vi "Byte Buffer.Write.Typed Double Array.vi"(0 "Byte Buffer in":refnum<class "Byte Buffer.lvclass">, 1 "data type":T1, 5 "buffer in":dbl[](array[numeric]), 7 "count":i64, 9 "buffer offset":u64, 11 "error in (no error)":errorcluster) -> (4 "Byte Buffer out":refnum<class "Byte Buffer.lvclass">, 6 "buffer out":dbl[](array[numeric]), 10 "new buffer offset":u64, 15 "error out":errorcluster)   [LabVIEW 2016, in "VeriStand Data.lvlib" / "Byte Buffer.lvclass"]
doc: "Reads <B>count</B> number of elements from the provided double float <B>buffer</B> and writes them to the <B>Byte Buffer</B> at the specified <B>buffer offset</B> and converted to the specified <B>data type</B>."
uses:
  Byte Buffer.lvclass
  Typedefs/Typedefs.Data Types.ctl
  Byte Buffer.lvclass/Byte Buffer.ctl
  Byte Buffer.Write (1D Boolean).vi
  Type Conversion/Type Conversion.From Double.Subset (1D Boolean).vi
  Byte Buffer.Write (1D SGL).vi
  Type Conversion/Type Conversion.From Double.Subset (1D SGL).vi
  Byte Buffer.Write (1D DBL).vi
  Byte Buffer.Write (1D I8).vi
  Type Conversion/Type Conversion.From Double.Subset (1D I8).vi
  Byte Buffer.Write (1D I16).vi
  Type Conversion/Type Conversion.From Double.Subset (1D I16).vi
  Byte Buffer.Write (1D I32).vi
  Type Conversion/Type Conversion.From Double.Subset (1D I32).vi
  Byte Buffer.Write (1D I64).vi
  Type Conversion/Type Conversion.From Double.Subset (1D I64).vi
  Byte Buffer.Write (1D U8).vi
  Type Conversion/Type Conversion.From Double.Subset (1D U8).vi
  Byte Buffer.Write (1D U16).vi
  Type Conversion/Type Conversion.From Double.Subset (1D U16).vi
  Byte Buffer.Write (1D U32).vi
  Type Conversion/Type Conversion.From Double.Subset (1D U32).vi
  Byte Buffer.Write (1D U64).vi
  Type Conversion/Type Conversion.From Double.Subset (1D U64).vi
  Byte Buffer.Write (String).vi
  Type Conversion/Type Conversion.From Double.vi
  Type Conversion/Type Conversion.From Double (1D Boolean).vi
  Type Conversion/Type Conversion.From Double (1D SGL).vi
  Type Conversion/Type Conversion.From Double (1D I8).vi
  Type Conversion/Type Conversion.From Double (1D I16).vi
  Type Conversion/Type Conversion.From Double (1D I32).vi
  Type Conversion/Type Conversion.From Double (1D I64).vi
  Type Conversion/Type Conversion.From Double (1D U8).vi
  Type Conversion/Type Conversion.From Double (1D U16).vi
  Type Conversion/Type Conversion.From Double (1D U32).vi
  Type Conversion/Type Conversion.From Double (1D U64).vi
  Byte Buffer.Subset.Set.vi
  Byte Buffer.Get Buffer Pointer.vi
  Byte Buffer.Get Buffer Size.vi
  Memory Management/Memory Management.MoveByteBlock.Read (String).vi
  Memory Management/Memory Management.Handle Return.vi
  Byte Buffer.Get Byte Order.vi
  VeriStand Data.lvlib
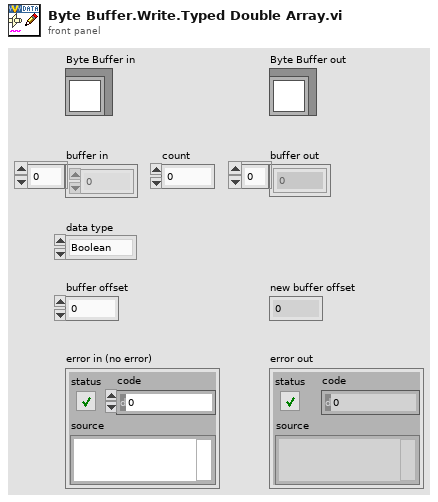
[diagram p1: front panel]
types:
  T1 = typedef "VeriStand Data.lvlib/Typedefs.Data Types.ctl" = enum16{"Boolean", "Single", "Double", "I8", "I16", "I32", "I64", "U8", "U16", "U32", "U64"}
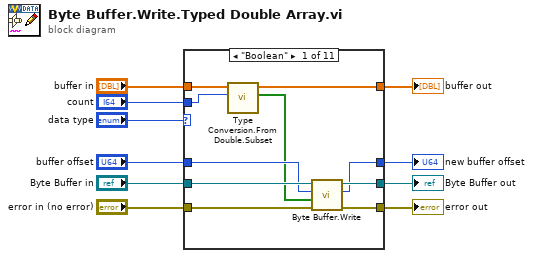
[diagram p0: block diagram]
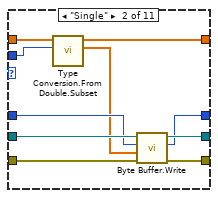
[diagram p2: hidden frame]
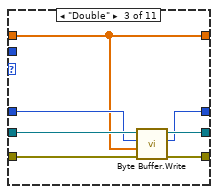
[diagram p3: hidden frame]
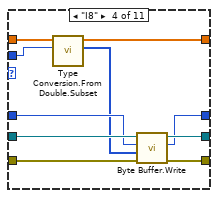
[diagram p4: hidden frame]
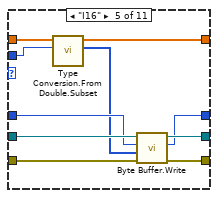
[diagram p5: hidden frame]
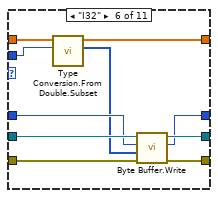
[diagram p6: hidden frame]
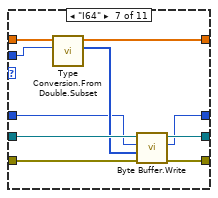
[diagram p7: hidden frame]
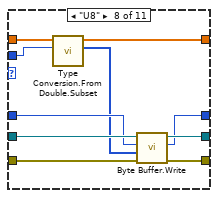
[diagram p8: hidden frame]
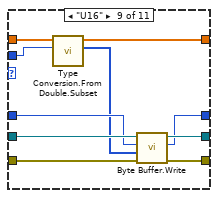
[diagram p9: hidden frame]
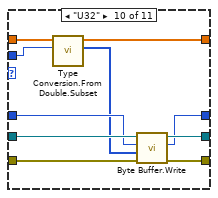
[diagram p10: hidden frame]
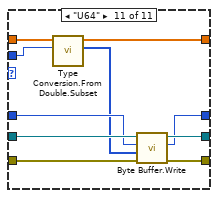
[diagram p11: hidden frame]
diagram:
  n1 = case shown="\"Boolean\"" "data type" {
    tunnel: "buffer in" -> [w20 w30 w32 w47 w57 w67 w77 w87 w97 w107 w117]
    tunnel: "buffer offset" -> [w17 w27 w35 w44 w54 w64 w69 w84 w94 w104 w114]
    tunnel: "Byte Buffer in" -> [w19 w29 w37 w46 w56 w66 w76 w86 w96 w106 w116]
    tunnel: [w18 w28 w36 w45 w55 w65 w75 w85 w95 w105 w115] -> w10
    tunnel: "error in (no error)" -> [w16 w26 w34 w43 w53 w63 w74 w83 w93 w103 w113]
    tunnel: [w15 w25 w33 w42 w52 w62 w73 w82 w92 w102 w112] -> w8
    tunnel: [w14 w24 w32 w41 w51 w61 w72 w81 w91 w101 w111] -> w6
    tunnel: "count" -> [w13 w23 _ w40 w50 w60 w71 w80 w90 w100 w110]
    tunnel: [w11 w21 w31 w38 w48 w58 w68 w78 w88 w98 w108] -> w2
    frame "Boolean" {
      n2 = call-poly "Type Conversion.From Double.Subset.vi"("count"=w13, "values in"=w20) -> ("converted values out"=w12:bool[], "values out"=w14:dbl[])  [unwired: 8 in]
      n3 = call-poly "Byte Buffer.Write.vi"("error in (no error)"=w16, "values"=w12, "buffer offset"=w17, "Byte Buffer in"=w19) -> ("error out"=w15:errorcluster, "new buffer offset"=w11:u64, "Byte Buffer out"=w18:refnum<class "Byte Buffer.lvclass">)  [unwired: 5 in]
    }
    frame "Single" {
      n4 = call-poly "Type Conversion.From Double.Subset.vi"("count"=w23, "values in"=w30) -> ("converted values out"=w22:sgl[], "values out"=w24:dbl[])  [unwired: 8 in]
      n5 = call-poly "Byte Buffer.Write.vi"("error in (no error)"=w26, "values"=w22, "buffer offset"=w27, "Byte Buffer in"=w29) -> ("error out"=w25:errorcluster, "new buffer offset"=w21:u64, "Byte Buffer out"=w28:refnum<class "Byte Buffer.lvclass">)  [unwired: 5 in]
    }
    frame "Double" {
      n6 = call-poly "Byte Buffer.Write.vi"("error in (no error)"=w34, "values"=w32, "buffer offset"=w35, "Byte Buffer in"=w37) -> ("error out"=w33:errorcluster, "new buffer offset"=w31:u64, "Byte Buffer out"=w36:refnum<class "Byte Buffer.lvclass">)  [unwired: 5 in]
    }
    frame "I8" {
      n7 = call-poly "Type Conversion.From Double.Subset.vi"("count"=w40, "values in"=w47) -> ("converted values out"=w39:i8[], "values out"=w41:dbl[])  [unwired: 8 in]
      n8 = call-poly "Byte Buffer.Write.vi"("error in (no error)"=w43, "values"=w39, "buffer offset"=w44, "Byte Buffer in"=w46) -> ("error out"=w42:errorcluster, "new buffer offset"=w38:u64, "Byte Buffer out"=w45:refnum<class "Byte Buffer.lvclass">)  [unwired: 5 in]
    }
    frame "I16" {
      n9 = call-poly "Type Conversion.From Double.Subset.vi"("count"=w50, "values in"=w57) -> ("converted values out"=w49:i16[], "values out"=w51:dbl[])  [unwired: 8 in]
      n10 = call-poly "Byte Buffer.Write.vi"("error in (no error)"=w53, "values"=w49, "buffer offset"=w54, "Byte Buffer in"=w56) -> ("error out"=w52:errorcluster, "new buffer offset"=w48:u64, "Byte Buffer out"=w55:refnum<class "Byte Buffer.lvclass">)  [unwired: 5 in]
    }
    frame "I32" {
      n11 = call-poly "Type Conversion.From Double.Subset.vi"("count"=w60, "values in"=w67) -> ("converted values out"=w59:i32[], "values out"=w61:dbl[])  [unwired: 8 in]
      n12 = call-poly "Byte Buffer.Write.vi"("error in (no error)"=w63, "values"=w59, "buffer offset"=w64, "Byte Buffer in"=w66) -> ("error out"=w62:errorcluster, "new buffer offset"=w58:u64, "Byte Buffer out"=w65:refnum<class "Byte Buffer.lvclass">)  [unwired: 5 in]
    }
    frame "I64" {
      n13 = call-poly "Type Conversion.From Double.Subset.vi"("count"=w71, "values in"=w77) -> ("converted values out"=w70:i64[], "values out"=w72:dbl[])  [unwired: 8 in]
      n14 = call-poly "Byte Buffer.Write.vi"("error in (no error)"=w74, "values"=w70, "buffer offset"=w69, "Byte Buffer in"=w76) -> ("error out"=w73:errorcluster, "new buffer offset"=w68:u64, "Byte Buffer out"=w75:refnum<class "Byte Buffer.lvclass">)  [unwired: 5 in]
    }
    frame "U8" {
      n15 = call-poly "Type Conversion.From Double.Subset.vi"("count"=w80, "values in"=w87) -> ("converted values out"=w79:u8[], "values out"=w81:dbl[])  [unwired: 8 in]
      n16 = call-poly "Byte Buffer.Write.vi"("error in (no error)"=w83, "values"=w79, "buffer offset"=w84, "Byte Buffer in"=w86) -> ("error out"=w82:errorcluster, "new buffer offset"=w78:u64, "Byte Buffer out"=w85:refnum<class "Byte Buffer.lvclass">)  [unwired: 5 in]
    }
    frame "U16" {
      n17 = call-poly "Type Conversion.From Double.Subset.vi"("count"=w90, "values in"=w97) -> ("converted values out"=w89:u16[], "values out"=w91:dbl[])  [unwired: 8 in]
      n18 = call-poly "Byte Buffer.Write.vi"("error in (no error)"=w93, "values"=w89, "buffer offset"=w94, "Byte Buffer in"=w96) -> ("error out"=w92:errorcluster, "new buffer offset"=w88:u64, "Byte Buffer out"=w95:refnum<class "Byte Buffer.lvclass">)  [unwired: 5 in]
    }
    frame "U32" {
      n19 = call-poly "Type Conversion.From Double.Subset.vi"("count"=w100, "values in"=w107) -> ("converted values out"=w99:u32[], "values out"=w101:dbl[])  [unwired: 8 in]
      n20 = call-poly "Byte Buffer.Write.vi"("error in (no error)"=w103, "values"=w99, "buffer offset"=w104, "Byte Buffer in"=w106) -> ("error out"=w102:errorcluster, "new buffer offset"=w98:u64, "Byte Buffer out"=w105:refnum<class "Byte Buffer.lvclass">)  [unwired: 5 in]
    }
    frame "U64" {
      n21 = call-poly "Type Conversion.From Double.Subset.vi"("count"=w110, "values in"=w117) -> ("converted values out"=w109:u64[], "values out"=w111:dbl[])  [unwired: 8 in]
      n22 = call-poly "Byte Buffer.Write.vi"("error in (no error)"=w113, "values"=w109, "buffer offset"=w114, "Byte Buffer in"=w116) -> ("error out"=w112:errorcluster, "new buffer offset"=w108:u64, "Byte Buffer out"=w115:refnum<class "Byte Buffer.lvclass">)  [unwired: 5 in]
    }
  }
  "error out" <- w8
  "Byte Buffer out" <- w10
  "new buffer offset" <- w2
  "buffer out" <- w6
